vi "ZH44044 multiAcq.vi"(5 "mAdr":u8=1 caption="从设备地址" min=1 max=250 format="%x", 7 "TestIndex":u8, 9 "num":u16=1 caption="寄存器个数/数值", 10 "regAdr":u16 caption="起始寄存器地址", 11 "FC":enum16{"读", "单个配置", "多个配置"}(ring) caption="功能码") -> (2 "values":dbl[](array[numeric]) caption="各通道值")   [LabVIEW 2015]
panel:
  out "data":string
  # "0,1,3,2,9,8,"
  # "airdry pump jet pump"
  # "11,10"
  # "onizer  5,6"
  # "7,"
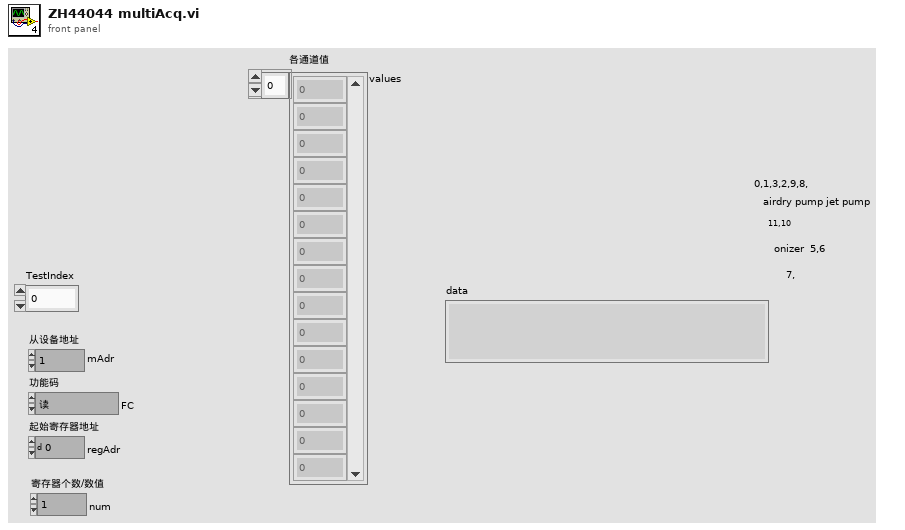
[diagram p1: front panel]
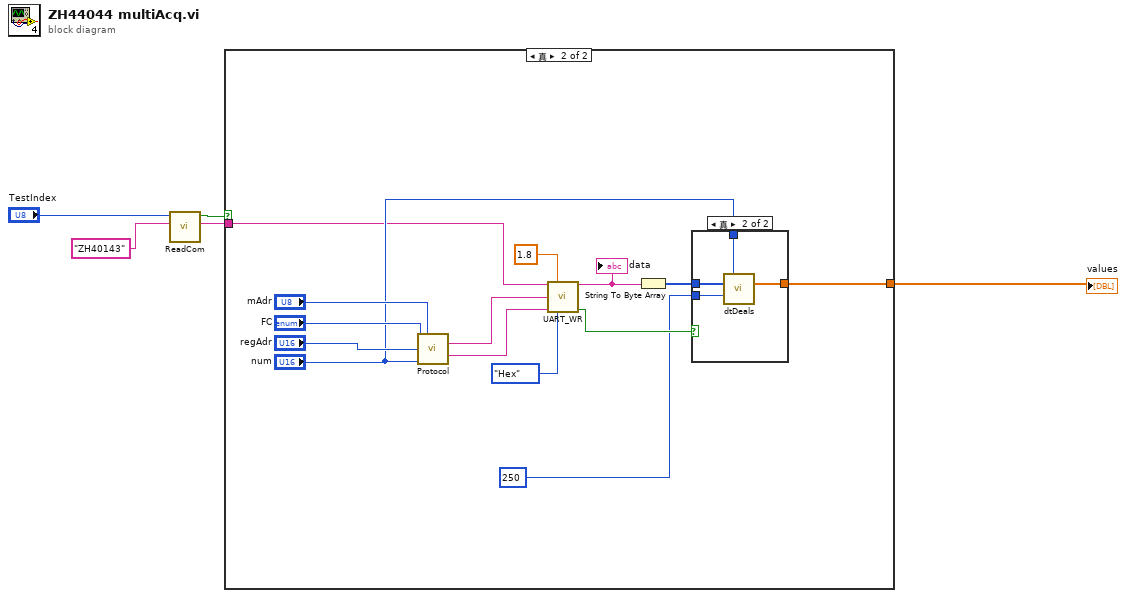
[diagram p0: block diagram]
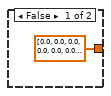
[diagram p2: hidden frame]
diagram:
  n1 = call "ReadCom.vi"("仪器名称"="ZH40143", "MyIndex"="TestIndex") -> ("COM"=w3:string, "OK?"=w1:bool)  [unwired: 7 in, 1 out]
  n2 = case shown="真" w1 {
    tunnel: [dbl[] [0.0, 0.0, 0.0, 0.0, 0.0, 0.0, 0.0, 0.0, 0.0, 0.0, 0.0, 0.0, 0.0, 0.0, 0.0, 0.0, 0.0, 0.0, 0.0, 0.0, 0.0, 0.0, 0.0, 0.0, 0.0, 0.0, 0.0, 0.0, 0.0, 0.0, 0.0, 0.0, 0.0, 0.0, 0.0, 0.0, 0.0, 0.0, 0.0, 0.0, 0.0, 0.0, 0.0, 0.0, 0.0, 0.0, 0.0, 0.0, 0.0, 0.0, 0.0, 0.0, 0.0, 0.0, 0.0, 0.0, 0.0, 0.0, 0.0, 0.0, 0.0, 0.0, 0.0, 0.0, 0.0, 0.0, 0.0, 0.0, 0.0, 0.0, 0.0, 0.0, 0.0, 0.0, 0.0, 0.0, 0.0, 0.0, 0.0, 0.0, 0.0] ("values") w9] -> w5
    tunnel: w3 -> [_ w7]
    frame False {
    }
    frame True {
      n3 = call "Protocol.vi"("FC"="FC", "mAdr"="mAdr", "regAdr"="regAdr", "num"="num") -> ("dtStr"=w17:string, "rdMatch"=w16:string)  [unwired: 10 in]
      n4 = call "UART_WR.vi"("coms"=w7, "timeOut_s"=1.8, "hexSend"=w17, "rdMatch"=w16, "strType"=enum16{"normal", "Hex"}."Hex") -> ("data"=w13:string, "OK"=w10:bool)  [unwired: 7 in, 2 out]
      "data" <- w13
      n5 = String To Byte Array(string=w13) -> (unsigned byte array=w12:u8[])
      n6 = case shown="真" w10 {
        tunnel: w12 -> [_ w24]
        tunnel: "num" -> [_ w23]
        tunnel: 250 ("rageMax") -> [_ w22]
        tunnel: [_ w21] -> w9
        frame False {
        }
        frame True {
          n7 = call "dtDeals.vi"("n"=w23, "inDts"=w24, "rageMax"=w22) -> ("values"=w21:dbl[])  [unwired: 12 in]
        }
      }
    }
  }
  "values" <- w5
